vi "readstringfromfile.vi"(9 "default value":string, 10 "Format string":string, 11 "Filename to read from:":path) -> (3 "output string":string)   [LabVIEW 2009]
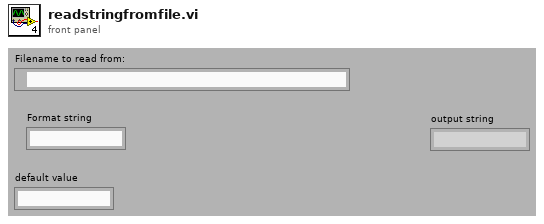
[diagram p1: front panel]
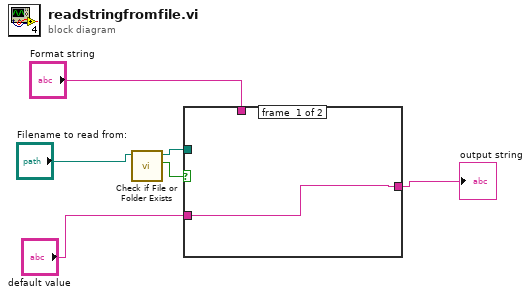
[diagram p0: block diagram]
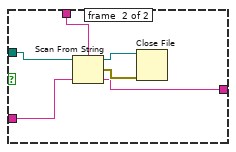
[diagram p2: hidden frame]
diagram:
  n1 = call <vilib>:"Check if File or Folder Exists.vi"("path"="Filename to read from:") -> ("file or folder exists?"=w5:bool, "dup path"=w3:path)  [unwired: 8 in, 1 out]
  n2 = case shown="False" w5 {
    tunnel: "default value" -> [w7 w12]
    tunnel: w3 -> [_ w13]
    tunnel: "Format string" -> [_ w11]
    tunnel: [w7 w8] -> w1
    frame #0 {
    }
    frame #1 {
      n3 = Scan From String(w11, w13, default 1=w12) -> (w10:refnum<file>, w9:errorcluster, output 1=w8:string)  [unwired: 1 in]
      n4 = Close File(refnum=w10, error in=w9) -> ()  [unwired: 2 out]
    }
  }
  "output string" <- w1
